vi "PatientDatabaseSearch.vi"(0 "Patient Info to Find":i32, 11 "file path (use dialog)":path=path "G:/Data/SUNYLymphNodeDB.txt") -> (1 "Last node of Last patient":i32, 2 "Node Set":string, 3 "Last Patient Number":i32, 6 "Last Node of Searched Patient":i32, 8 "Searched Node Location":T2, 10 "Node Classification Of Searched":T1(ring), 12 "Tissue Type of Last Node":T2, 13 "Tissue Location (Other)":string, 14 "Node Classification Of Last Patient":T1(ring), 15 "Fresh?":bool)   [LabVIEW 2022 SP3]
uses:
  <vilib>/regexp/Match Regular Expression.xnode
  ViewData/-ReadEye/TypeDefs/TissueType.ctl
panel:
  out "Node Number":i32[](array[numeric])
  out "Patient number":i32[](array[numeric])
  out "error out":errorcluster
  out "Node Location":string[](array[string])
  out "Node Class":string[](array[string])
  out "File Name":string[](array[string])
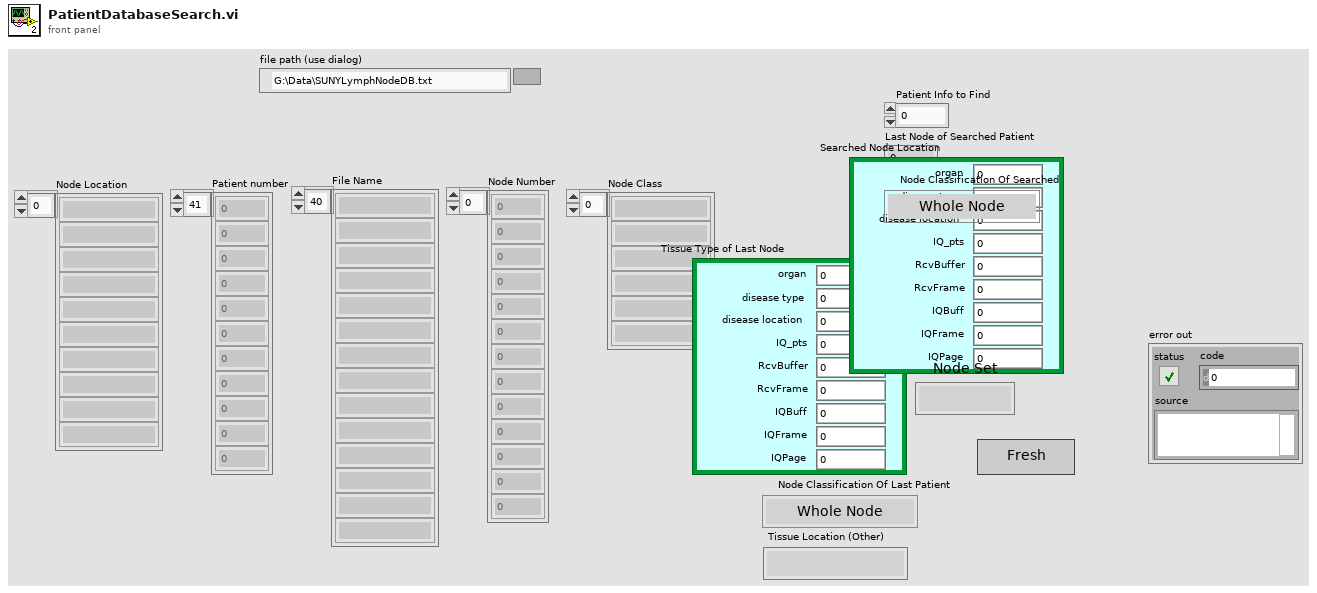
[diagram p1: front panel]
types:
  T1 = enum16{"Whole Node", "Sentinel A", "Sentinel B", "Sentinel C"}
  T2 = typedef "TissueType.ctl" = cluster{"organ":i16, "disease type":i16, "disease location":i16, "IQ_pts":u16, "RcvBuffer":u8, "RcvFrame":u16, "IQBuff":u8, "IQFrame":u16, "IQPage":u8}
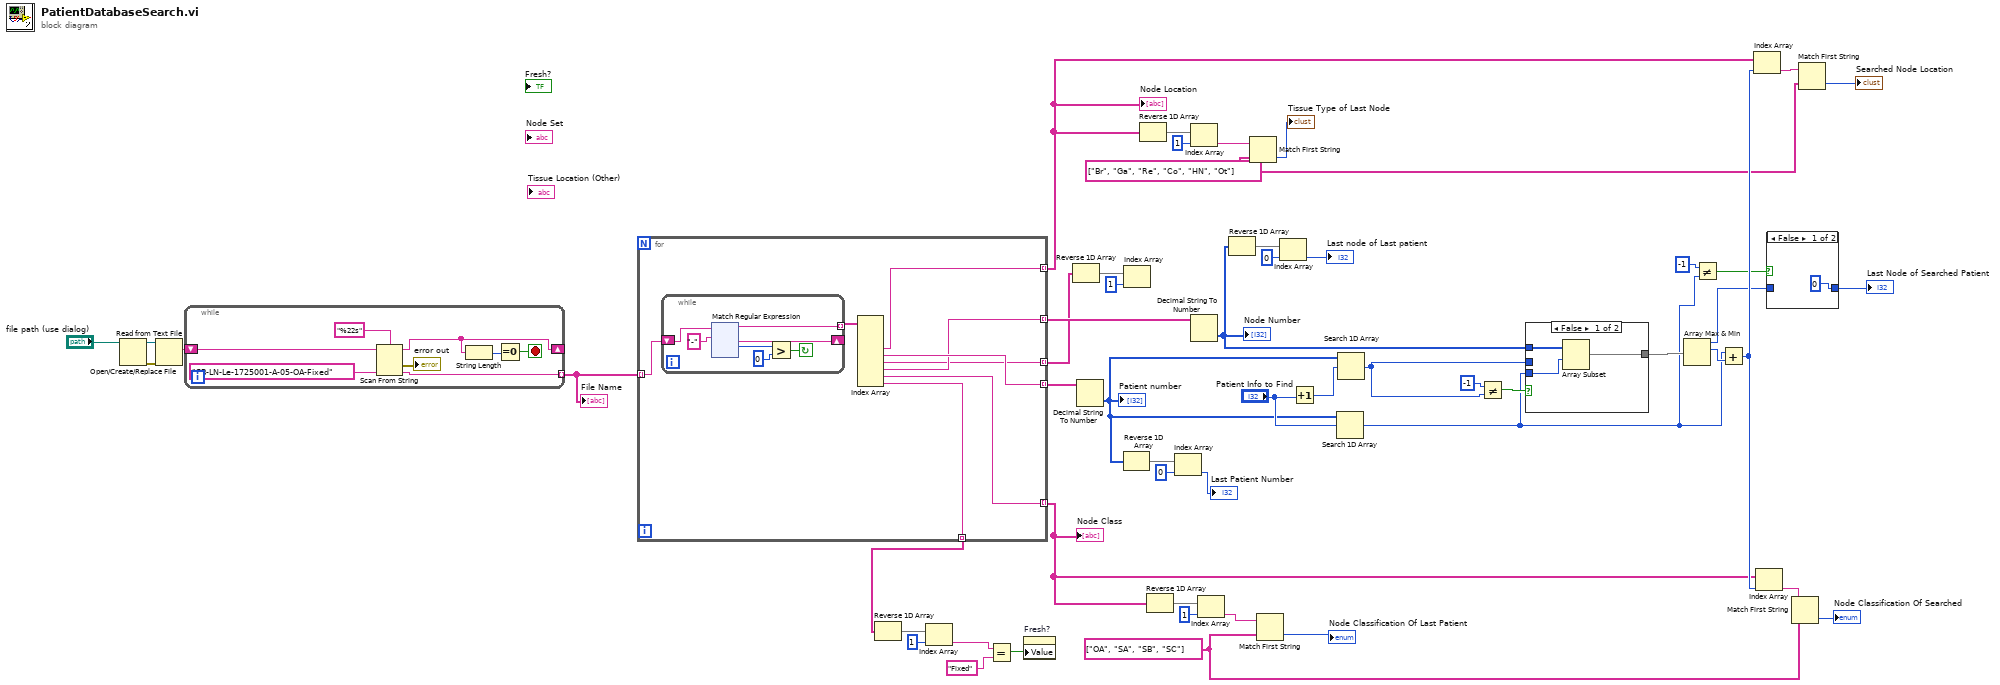
[diagram p0: block diagram]
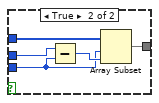
[diagram p3: hidden frame]
diagram:
  w14 = string[] ["Br", "Ga", "Re", "Co", "HN", "Ot"] ("string array")
  w10 = string[] ["OA", "SA", "SB", "SC"] ("string array")
  n1 = Open/Create/Replace File(file path (use dialog)="file path (use dialog)") -> (refnum out=w52:refnum<file>, error out=w51:errorcluster)  [unwired: 5 in, 1 out]
  n2 = Read from Text File(file (use dialog)=w52, error in=w51) -> (text=w50:string)  [unwired: 2 in, 3 out]
  n3 = while {
    tunnel: [w60] -> w49 mode=indexing
    shift-right: [w56] -> _
    shift-left: w50 -> [w61]
    stop <- w58 stop-if-true
    n4 = Scan From String(format string="%22s", input string=w61, default 1="SB-LN-Le-1725001-A-05-OA-Fixed" ("default value 1")) -> (remaining string=w56:string, error out=→"error out":errorcluster, output 1=w60:string)  [unwired: 2 in, 1 out]
    n5 = String Length(string=w56) -> (length=w59:i32)
    n6 = Equal To 0?(x=w59) -> (x = 0?=w58:bool)
  }
  "File Name" <- w49
  n7 = for {
    tunnel: [w67] -> w32 mode=indexing
    tunnel: [w65] -> w47 mode=indexing
    tunnel: [w64] -> w33 mode=indexing
    tunnel: [w66] -> w48 mode=indexing
    tunnel: w49 -> [w69] mode=indexing
    tunnel: [w63] -> w4 mode=indexing
    tunnel: [w62] -> w7 mode=indexing
    n8 = while {
      tunnel: [w71] -> w68 mode=indexing
      shift-right: [w70] -> _
      shift-left: w69 -> [w76]
      stop <- w73 continue-if-true
      n9 = xnode "Match Regular Expression"("input string"=w76, "regular expression"="-") -> ("before match"=w71:string, "after match"=w70:string, "offset past match"=w74:i32)  [unwired: 4 in, 2 out]
      n10 = Greater?(x=w74, y=0) -> (0:w73:bool)
    }
    n11 = Index Array(array=w68) -> (element #3=w67:string, element #4=w66:string, element #5=w62:string, element #6=w65:string, element #7=w64:string, element #8=w63:string)  [unwired: 8 in, 2 out]
  }
  "Node Class" <- w33
  "Node Location" <- w32
  n12 = Reverse 1D Array(array=w4) -> (reversed array=w6:string[])
  n13 = Index Array(array=w6, index=1) -> (element=w3:string)
  n14 = Equal?(x=w3, y="Fixed") -> (x = y?=w1:bool)
  n15 = property on="Fresh?" class="Bool (strict)"("Value"=w1) -> ()  [unwired: 2 in, 2 out]
  n16 = Reverse 1D Array(array=w7) -> (reversed array=w9:string[])
  n17 = Decimal String To Number(string=w48) -> (number=w22:i32[])  [unwired: 2 in, 1 out]
  "Patient number" <- w22
  n18 = Reverse 1D Array(array=w22) -> (reversed array=w23:i32[])
  n19 = Index Array(array=w9, index=1) -> ()  [unwired: 1 out]
  n20 = Reverse 1D Array(array=w32) -> (reversed array=w27:string[])
  n21 = Reverse 1D Array(array=w33) -> (reversed array=w29:string[])
  n22 = Index Array(array=w23, index=0) -> (element=→"Last Patient Number":i32)
  n23 = Index Array(array=w27, index=1) -> (element=w28:string)
  n24 = Decimal String To Number(string=w47) -> (number=w17:i32[])  [unwired: 2 in, 1 out]
  "Node Number" <- w17
  n25 = Index Array(array=w29, index=1) -> (element=w30:string)
  n26 = Reverse 1D Array(array=w17) -> (reversed array=w19:i32[])
  n27 = Match First String(2:w14, 3:w28) -> (0:→"Tissue Type of Last Node":i32)  [unwired: 1 out]
  n28 = Match First String(2:w10, 3:w30) -> (0:→"Node Classification Of Last Patient":i32)  [unwired: 1 out]
  n29 = Index Array(array=w19, index=0) -> (element=→"Last node of Last patient":i32)
  n30 = Increment(x="Patient Info to Find") -> (x+1=w45:i32)
  n31 = Search 1D Array(1D array=w22, element="Patient Info to Find") -> (index of element=w34:i32)  [unwired: 1 in]
  n32 = Search 1D Array(1D array=w22, element=w45) -> (index of element=w44:i32)  [unwired: 1 in]
  n33 = Not Equal?(x=-1, y=w44) -> (x != y?=w43:bool)
  n34 = case shown="False" w43 {
    tunnel: [w196 w199] -> w40
    tunnel: w44 -> [_ w201]
    tunnel: w34 -> [w195 w197]
    tunnel: w17 -> [w194 w198]
    frame False {
      n35 = Array Subset(array=w194, index=w195) -> (w196:i32[])  [unwired: 1 in]
    }
    frame True {
      n36 = Subtract(x=w201, y=w197) -> (x-y=w200:i32)
      n37 = Array Subset(array=w198, index=w197, length=w200) -> (w199:i32[])
    }
  }
  n38 = Array Max & Min(array=w40) -> (max value=w38:i32, max index (indices)=w39:i32)  [unwired: 2 out]
  n39 = Not Equal?(x=-1, y=w34) -> (x != y?=w36:bool)
  n40 = Add(x=w34, y=w39) -> (x+y=w41:i32)
  n41 = Index Array(array=w32, index=w41) -> (element=w15:string)
  n42 = Index Array(array=w33, index=w41) -> (element=w12:string)
  n43 = case shown="False" w36 {
    tunnel: w38 -> [_ w203]
    tunnel: [0 w203] -> w37
    frame False {
    }
    frame True {
    }
  }
  "Last Node of Searched Patient" <- w37
  n44 = Match First String(2:w10, 3:w12) -> (0:→"Node Classification Of Searched":i32)  [unwired: 1 out]
  n45 = Match First String(2:w14, 3:w15) -> (0:→"Searched Node Location":i32)  [unwired: 1 out]
